vi "AlliGator Find & Plot Threshold Crossing Position.vi"(6 "Threshold":dbl, 8 "Error In":errorcluster, 9 "Time Stamp":dbl, 10 "Lifetime Graph":refnum<vi>, 11 "Decay Graph":refnum<vi>) -> (0 "Error Out":errorcluster, 3 "Crossing Position":dbl)   [LabVIEW 2021, in "AlliGator Decay Preprocessing.lvlib"]
doc: "Find the location where the decay reaches the provided thresholf (from below), returns that position and adds it to the last plot in the <B>Lifetime & Other Parameters Graph</B>."
uses:
  AlliGator Decay Preprocessing.lvlib
  Graphs/XY Graph/XY Graph Add-Ons.lvlib
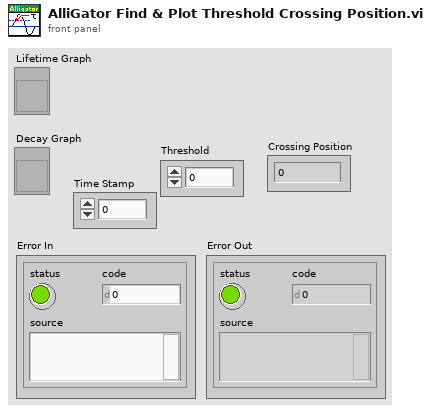
[diagram p1: front panel]
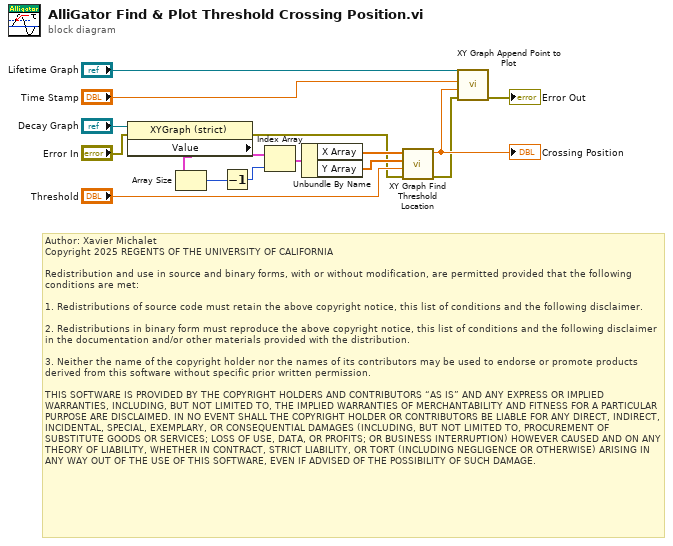
[diagram p0: block diagram]
diagram:
  # "Author: Xavier Michalet\nCopyright 2025 REGENTS OF THE UNIVERSITY OF CALIFORNIA\n\nRedistribution and use in source and binary forms, with or without modification, are permitted provided that the following conditions are met:\n\n1. Redistributions of source code must retain the above copyright notice, this list of conditions and the following disclaimer.\n\n2. Redistributions in binary form must reproduce the above copyright notice, this list of conditions and the following disclaimer in the documentation and/or other materials provided with the distribution.\n\n3. Neither the name of the copyright holder nor the names of its contributors may be used to endorse or promote products derived from this software without specific prior written permission.\n\nTHIS SOFTWARE IS PROVIDED BY THE COPYRIGHT HOLDERS AND CONTRIBUTORS “AS IS” AND ANY EXPRESS OR IMPLIED WARRANTIES, INCLUDING, BUT NOT LIMITED TO, THE IMPLIED WARRANTIES OF MERCHANTABILITY AND FITNESS FOR A PARTICULAR PURPOSE ARE DISCLAIMED. IN NO EVENT SHALL THE COPYRIGHT HOLDER OR CONTRIBUTORS BE LIABLE FOR ANY DIRECT, INDIRECT, INCIDENTAL, SPECIAL, EXEMPLARY, OR CONSEQUENTIAL DAMAGES (INCLUDING, BUT NOT LIMITED TO, PROCUREMENT OF SUBSTITUTE GOODS OR SERVICES; LOSS OF USE, DATA, OR PROFITS; OR BUSINESS INTERRUPTION) HOWEVER CAUSED AND ON ANY THEORY OF LIABILITY, WHETHER IN CONTRACT, STRICT LIABILITY, OR TORT (INCLUDING NEGLIGENCE OR OTHERWISE) ARISING IN ANY WAY OUT OF THE USE OF THIS SOFTWARE, EVEN IF ADVISED OF THE POSSIBILITY OF SUCH DAMAGE."
  n1 = property class="XYGraph (strict)"(reference="Decay Graph", error in="Error In") -> (error out=w2:errorcluster, "Value"=w13:cluster{"X Array":dbl[], "Y Array":dbl[]}[])  [unwired: 1 out]
  n2 = Array Size(array=w13) -> (size(s)=w12:i32)
  n3 = Decrement(x=w12) -> (x-1=w8:i32)
  n4 = Index Array(array=w13, index=w8) -> (element=w11:cluster{"X Array":dbl[], "Y Array":dbl[]})
  n5 = Unbundle By Name(w11) -> ("X Array"=w6:dbl[], "Y Array"=w4:dbl[])
  n6 = call "XY Graph Find Threshold Location.vi"("Error In"=w2, "Threshold"="Threshold", "Y Array"=w4, "X Array"=w6) -> ("Error Out"=w1:errorcluster, "Threshold Location"=w5:dbl)  [unwired: 5 in, 1 out]
  "Crossing Position" <- w5
  n7 = call "XY Graph Append Point to Plot.vi"("error in (no error)"=w1, "y"=w5, "x"="Time Stamp", "XYGraph in"="Lifetime Graph") -> ("error out"=→"Error Out":errorcluster)  [unwired: 4 in, 3 out]
